vi "Suite.vi"(8 "error in (no error)":errorcluster, 10 "LUnit Test Suite in":refnum<class "LUnit Test Suite.lvclass">, 11 "LUnit Test Case In":refnum<class "LUnit Test Case.lvclass">) -> (0 "error out":errorcluster, 2 "LUnit Test Suite Out":refnum<class "LUnit Test Suite.lvclass">, 3 "LUnit Test Case Out":refnum<class "LUnit Test Case.lvclass">)   [LabVIEW 2020, in "LUnit Test Case.lvclass"]
doc: "Factory method to generate a Test Suite object for the test case class.\nThe Test Suite input is used as a collecting parameter to which the test case methods are appended. This can be useful when using custom test suite classes."
uses:
  LUnit Test Case.lvclass
  C:/git/astemes-lunit/source/Runnable.lvclass
  LUnit Test Suite.lvclass
  LUnit Test Case.lvclass/LUnit Test Case.ctl
  C:/git/astemes-lunit/source/LUnit Test Case.lvclass
  Framework/Utilities/Utilities.lvlib
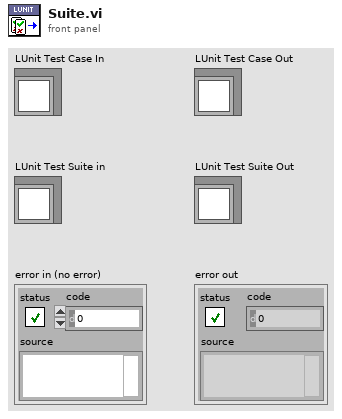
[diagram p1: front panel]
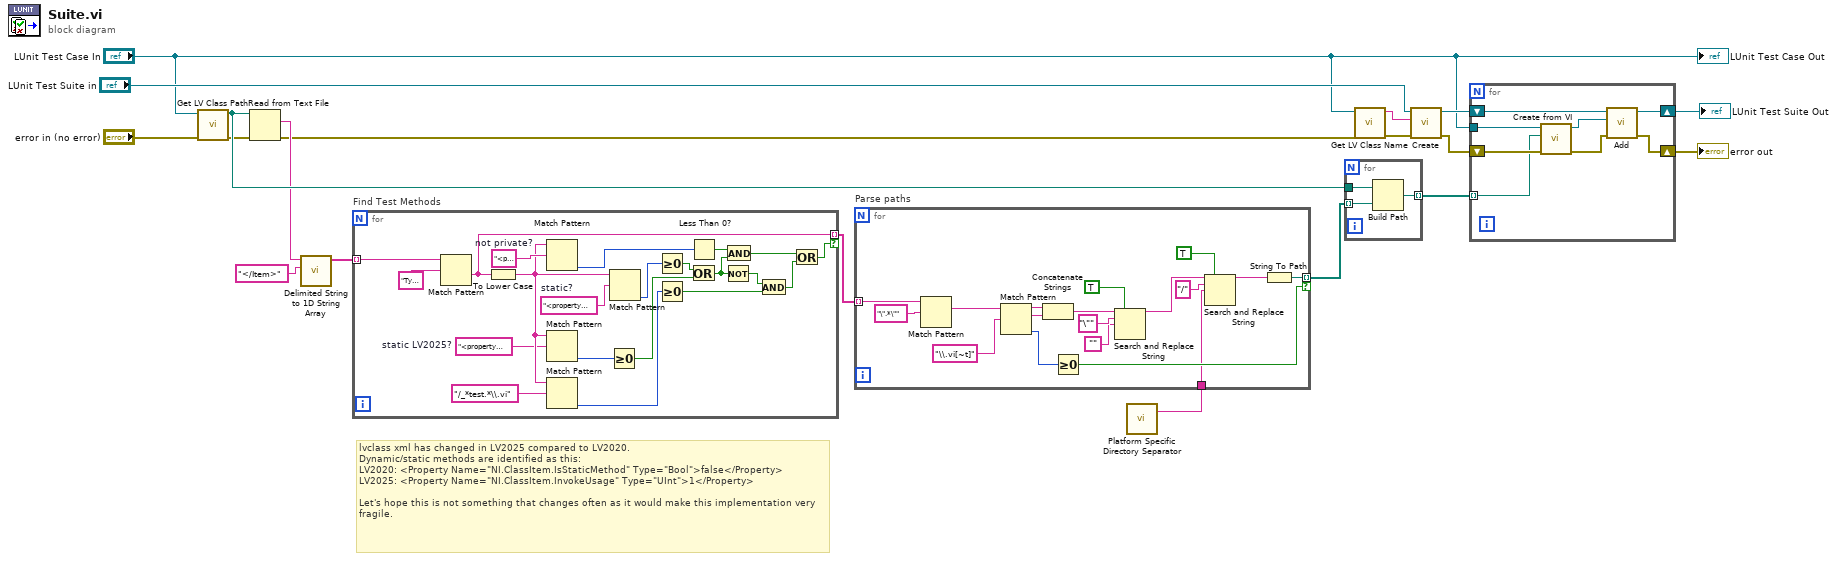
[diagram p0: block diagram]
diagram:
  # "lvclass xml has changed in LV2025 compared to LV2020.\nDynamic/static methods are identified as this:\nLV2020: <Property Name=\"NI.ClassItem.IsStaticMethod\" Type=\"Bool\">false</Property>\nLV2025: <Property Name=\"NI.ClassItem.InvokeUsage\" Type=\"UInt\">1</Property>\n\nLet's hope this is not something that changes often as it would make this implementation very fragile."
  n1 = call <vilib>:"Get LV Class Path.vi"("error in (no error)"="error in (no error)", "object"="LUnit Test Case In") -> ("error out"=w3:errorcluster, "class path"=w10:path)  [unwired: 8 in]
  n2 = Read from Text File(file (use dialog)=w10, error in=w3) -> (text=w4:string, error out=w2:errorcluster)  [unwired: 2 in, 2 out]
  n3 = call <vilib>:"Delimited String to 1D String Array.vi"("delimiter"="</Item>" ("regular expression"), "delimited string"=w4) -> ("string array"=w8:string[])  [unwired: 9 in]
  n4 = for "Find Test Methods" {
    tunnel: w8 -> [w40] mode=indexing
    tunnel: [w36] -> w7 mode=indexing if=w28
    w23 = "<property name=\"ni.classitem.invokeusage\" type=\"uint\">0"  # static LV2025?
    w35 = "<property name=\"ni.classitem.methodscope\" type=\"uint\">2"  # not private?
    w39 = "<property name=\"ni.classitem.isstaticmethod\" type=\"bool\">true"  # static?
    n5 = Match Pattern(string=w40, regular expression="Type=\"VI\"") -> (after substring=w36:string)  [unwired: 1 in, 3 out]
    n6 = To Lower Case(string=w36) -> (all lower case string=w24:string)
    n7 = Match Pattern(string=w24, regular expression=w35) -> (offset past match=w37:i32)  [unwired: 1 in, 3 out]
    n8 = Match Pattern(string=w24, regular expression=w23) -> (offset past match=w25:i32)  [unwired: 1 in, 3 out]
    n9 = Match Pattern(string=w24, regular expression="/_*test.*\\.vi") -> (offset past match=w32:i32)  [unwired: 1 in, 3 out]
    n10 = Greater Or Equal To 0?(x=w25) -> (x >= 0?=w21:bool)
    n11 = Match Pattern(string=w24, regular expression=w39) -> (offset past match=w38:i32)  [unwired: 1 in, 3 out]
    n12 = Greater Or Equal To 0?(x=w38) -> (x >= 0?=w31:bool)
    n13 = Greater Or Equal To 0?(x=w32) -> (x >= 0?=w29:bool)
    n14 = Less Than 0?(x=w37) -> (x < 0?=w34:bool)
    n15 = Or(x=w31, y=w21) -> (x .or. y?=w22:bool)
    n16 = Not(x=w22) -> (.not. x?=w30:bool)
    n17 = And(x=w34, y=w22) -> (x .and. y?=w27:bool)
    n18 = And(x=w30, y=w29) -> (x .and. y?=w26:bool)
    n19 = Or(x=w27, y=w26) -> (x .or. y?=w28:bool)
  }
  n20 = call "Platform Specific Directory Separator.vi"() -> ("Directory separator"=w1:string)  [unwired: 4 in]
  n21 = for "Parse paths" {
    tunnel: w7 -> [w58] mode=indexing
    tunnel: [w53] -> w5 mode=indexing if=w44
    tunnel: w1 -> [w41]
    n22 = Match Pattern(string=w58, regular expression="\".*\"") -> (match substring=w47:string)  [unwired: 1 in, 3 out]
    n23 = Match Pattern(string=w47, regular expression="\\.vi[~t]") -> (before substring=w49:string, match substring=w48:string, offset past match=w45:i32)  [unwired: 1 in, 1 out]
    n24 = Concatenate Strings(w49, w48) -> (w46:string)
    n25 = Greater Or Equal To 0?(x=w45) -> (x >= 0?=w44:bool)
    n26 = Search and Replace String(replace all?=TRUE ("replace all? (F)"), input string=w46, search string="\"", replace string="") -> (result string=w52:string)  [unwired: 4 in, 3 out]
    n27 = Search and Replace String(replace all?=TRUE ("replace all? (F)"), input string=w52, search string="/", replace string=w41) -> (result string=w51:string)  [unwired: 4 in, 3 out]
    n28 = String To Path(string=w51) -> (path=w53:path)
  }
  n29 = for {
    tunnel: w10 -> [w61]
    tunnel: w5 -> [w60] mode=indexing
    tunnel: [w59] -> w9 mode=indexing
    n30 = Build Path(base path=w61, name or relative path=w60) -> (appended path=w59:path)
  }
  n31 = call <vilib>:"Get LV Class Name.vi"("error in (no error)"=w2, "object"="LUnit Test Case In") -> ("error out"=w11:errorcluster, "class name"=w12:string)  [unwired: 8 in]
  n32 = call "Create.vi"("error in (no error)"=w11, "Suite Name"=w12, "LUnit Test Suite in"="LUnit Test Suite in") -> ("error out"=w18:errorcluster, "LUnit Test Suite Out"=w19:refnum<class "LUnit Test Suite.lvclass">)  [unwired: 7 in]
  n33 = for {
    tunnel: w9 -> [w62] mode=indexing
    shift-right: [w68] -> w17
    shift-left: w19 -> [w69]
    shift-right: [w66] -> w15
    shift-left: w18 -> [w65]
    tunnel: "LUnit Test Case In" -> [w63]
    n34 = call "Create from VI.vi"("error in (no error)"=w65, "Test Method VI Path"=w62, "LUnit Test Case In"=w63) -> ("error out"=w67:errorcluster, "LUnit Test Case Out"=w64:refnum<class "LUnit Test Case.lvclass">)  [unwired: 7 in]
    n35 = call "Add.vi"("error in (no error)"=w67, "Runnable"=w64, "LUnit Test Suite In"=w69) -> ("error out"=w66:errorcluster, "LUnit Test Suite Out"=w68:refnum<class "LUnit Test Suite.lvclass">)  [unwired: 7 in]
  }
  "error out" <- w15
  "LUnit Test Suite Out" <- w17
  "LUnit Test Case Out" <- "LUnit Test Case In"
